vi "Test.vi"() -> ()   [LabVIEW 2013]
uses:
  Controls/PID parameters.ctl
panel:
  out "PID Speed =0?":bool
  in  "Live Load":dbl min=-200.0 max=200.0 format="%_4g"
  in  "Target Load":dbl
  in  "Load Speed":dbl
  in  "PID":T1={"Kp"=0.0, "Kd"=0.04, "Ki"=0.005001} {"Ki" min=0.0 max=200.0 format="%.6f"; "Kd" min=0.0 max=200.0 format="%.6f"; "Kp" min=0.0 max=200.0 format="%.6f"}
  out "Out Speed":dbl
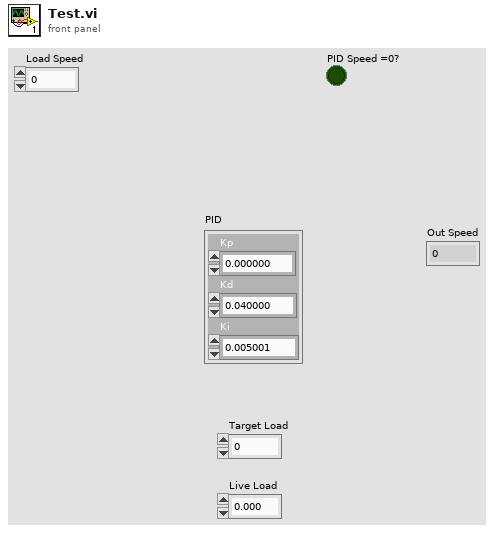
[diagram p1: front panel]
types:
  T1 = typedef "PID parameters.ctl" = cluster{"Kp":dbl, "Kd":dbl, "Ki":dbl}
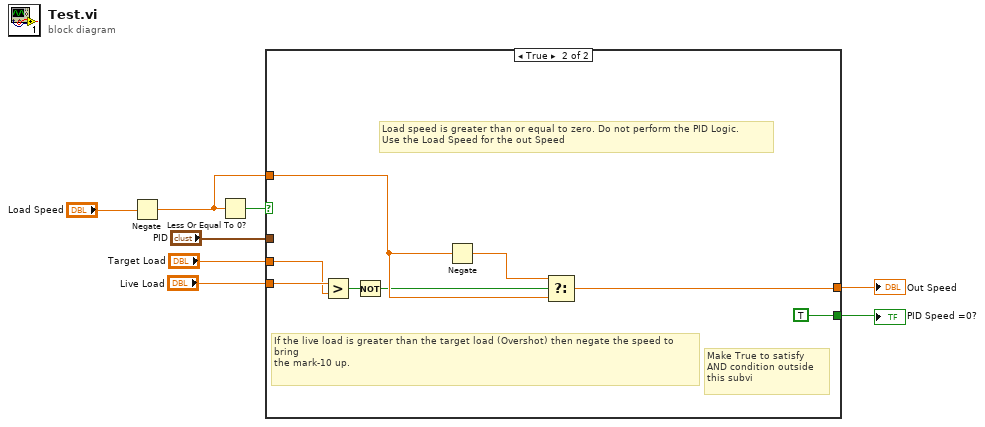
[diagram p0: block diagram]
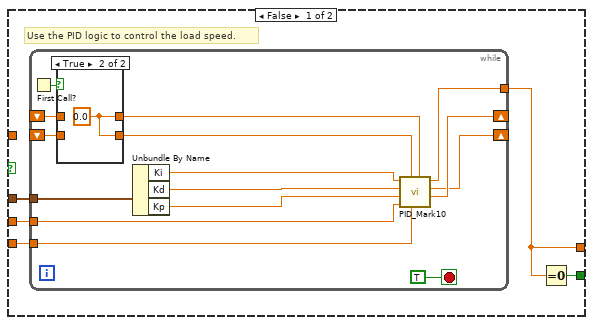
[diagram p2: hidden frame]
diagram:
  n1 = Negate(x="Load Speed") -> (-x=w1:dbl)
  n2 = Less Or Equal To 0?(x=w1) -> (x <= 0?=w4:bool)
  n3 = case shown="True" w4 {
    tunnel: [w9 w35] -> w8
    tunnel: w1 -> [_ w36]
    tunnel: "Target Load" -> [w13 w38]
    tunnel: "Live Load" -> [w12 w39]
    tunnel: "PID" -> [w11 _]
    tunnel: [w10 TRUE] -> w3
    frame False {
      # "Use the PID logic to control the load speed."
      n4 = while {
        tunnel: [w17] -> w9
        shift-right: [w25] -> _
        shift-left: _ -> [w26]
        shift-right: [w22] -> _
        shift-left: _ -> [w23]
        tunnel: w11 -> [w20]
        tunnel: w13 -> [w15]
        tunnel: w12 -> [w14]
        stop <- TRUE stop-if-true
        n5 = First Call?() -> (First Call?: T/F=w28:bool)
        n6 = case shown="True" w28 {
          tunnel: [w30 w31] -> w27
          tunnel: w26 -> [w30 _]
          tunnel: [w29 w31] -> w24
          tunnel: w23 -> [w29 _]
          frame False {
          }
          frame True {
            w31 = 0.0 ("Error Previous")
          }
        }
        n7 = Unbundle By Name(w20) -> ("Ki"=w16:dbl, "Kd"=w18:dbl, "Kp"=w19:dbl)
        n8 = call "PID_Mark10.vi"("Error Previous"=w27, "Input"=w14, "Error Accumulator"=w24, "Setpoint"=w15, "Kp"=w19, "Kd"=w18, "Ki"=w16) -> ("Error Previous"=w25:dbl, "Error Accumulator"=w22:dbl, "Drive out"=w17:dbl)  [unwired: 2 in]
      }
      n9 = Equal To 0?(x=w9) -> (x = 0?=w10:bool)
    }
    frame True {
      # "Make True to satisfy\nAND condition outside\nthis subvi"
      # "If the live load is greater than the target load (Overshot) then negate the speed to bring\nthe mark-10 up."
      # "Load speed is greater than or equal to zero. Do not perform the PID Logic. \nUse the Load Speed for the out Speed"
      n10 = Greater?(x=w39, y=w38) -> (0:w33:bool)
      n11 = Not(x=w33) -> (.not. x?=w32:bool)
      n12 = Negate(x=w36) -> (-x=w37:dbl)
      n13 = Select(t=w37, s=w32, f=w36) -> (s? t:f=w35:dbl)
    }
  }
  "Out Speed" <- w8
  "PID Speed =0?" <- w3
